vi "Dashboard Main.vi"() -> ()   [LabVIEW 2012]
uses:
  <vilib>/event_ctls.llb/eventvkey.ctl
  <vilib>/Utility/config.llb/Read Key (String).vi
  <vilib>/Utility/config.llb/Read Key (I32).vi
  <vilib>/Utility/config.llb/Write Key (String).vi
  <vilib>/Utility/config.llb/Write Key (I32).vi
  <vilib>/Utility/config.llb/NI_LVConfig.lvlib
panel:
  out "Mode":T1(ring)=enum."Auto Disabled"
  in  "Viewer":enum32{"Camera Image", "Variables"}(tab)
  out "Mbps":dbl format="%#.1g"
  in  "Enable":bool=TRUE
  in  "DB Camera Config":bool
  out "Mbps":bool
  out "fps":dbl format="%#.1g"
  out "Image Error Message":string="Timeout in Camera Communications"
  out "Camera Image":T2(plugin-control)
  out "Camera Image 2":T2(plugin-control)
  in  "Camera Settings":T3={"Frame Rate"=15, "Compression"=30, "Size"=1} {"Frame Rate" scale=1.0..30.0; "Size" items=["640x480", "320x240", "160x120"]}
  out "Camera IP 2":string
  out "Camera IP":string
  out "fps 2":dbl format="%#.1g"
  out "Mbps 2":dbl format="%#.1g"
  in  "Enable 2":bool=TRUE
  in  "FR":i32=15
  out "Tree":string(tree)
  in  "Dashboard Tab":enum32{"Operation", "Test", "Checklist"}(tab)
  in  "Slider":dbl(slide) scale=0.0..100.0 scale format="%#_3g"
  in  "On/Off":bool caption="Solenoid"
  in  "Test Name":u16(ring) items=["Select the test to run...", "Example Test", "-------------------------------", "List of tests is built in robot code.", "Replace with your own automated tests."]
  in  "Test Tree":string(tree)
  in  "Motor":cluster{"Value":dbl, "Enable":bool} {"Value" scale=-1.0..1.0 scale format="%#_3g"}
  out "Progress":T4 {"Test Progress" scale=0.0..100.0}
  in  "Rev/Fwd":cluster{"Forward":bool, "Reverse":bool}
  in  "Ring":u16(ring) items=["Auto", "Fixed indoor", "Fixed outdoor 1", "Fixed outdoor 2", "Fixed fluorescent 1", "Fixed fluorescent 2", "Hold current"]
  in  "Listbox":i32(listbox)
  out "Robot IP":string
  out "Battery Value":dbl(slide) scale=0.0..14.0 scale format="%#_2e"
  out "Battery":sgl(graph)
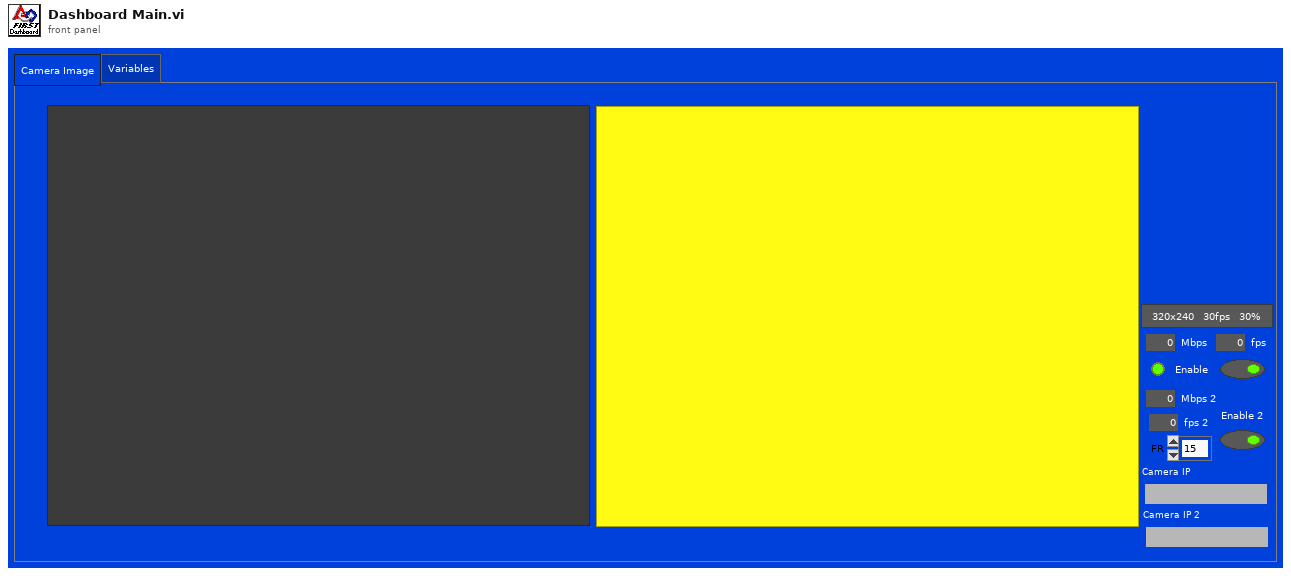
[diagram p1: front panel]
types:
  T1 = enum8{"Tele-Op Disabled", "Tele-Op Enabled", "Auto Disabled", "Auto Enabled", "Test Disabled", "Test Enabled", ""}
  T2 = typedef "IMAQ Image.ctl" = refnum<image>
  T3 = cluster{"Frame Rate":i32, "Compression":i32, "Size":u16}
  T4 = cluster{"Test Progress":u8, "Test Progress Text":string}
  T5 = typedef "Image Type" = u32
  T6 = cluster{"Competition mode":bool, "Robot Link":bool, "Autonomous":bool, "Enabled":bool, "E-Stop":bool, "Simulated":bool, "TestMode":bool, "Docked Window":bool}
  T7 = typedef "LVRectTypeDef.ctl" = cluster{"Left":i16, "Top":i16, "Right":i16, "Bottom":i16}
  T8 = typedef "NI_LVConfig.lvlib/Config Data RefNum.ctl" = refnum<k1>
  T9 = typedef "eventvkey.ctl" = enum16{"ASCII", "Enter", "Return", "Shift", "Ctrl", "Alt", "Cmd", "Opt", "Caps", "NumLock", "Clear", "Break", "Up", "Down", "Left", "Right", "Insert", "Delete", "Home", "End", "PageUp", "PageDown", "Escape", "Help", "Pause", "ScrollLock", "F1", "F2", "F3", "F4", "F5", "F6", "F7", "F8", "F9", "F10", "F11", "F12", "F13", "F14", "F15", "F16", "F17", "F18", "F19", "F20", "F21", "F22", "F23", "F24", "Play", "VolumeUp", "VolumeDown", "Mute", "Two Byte Char"}
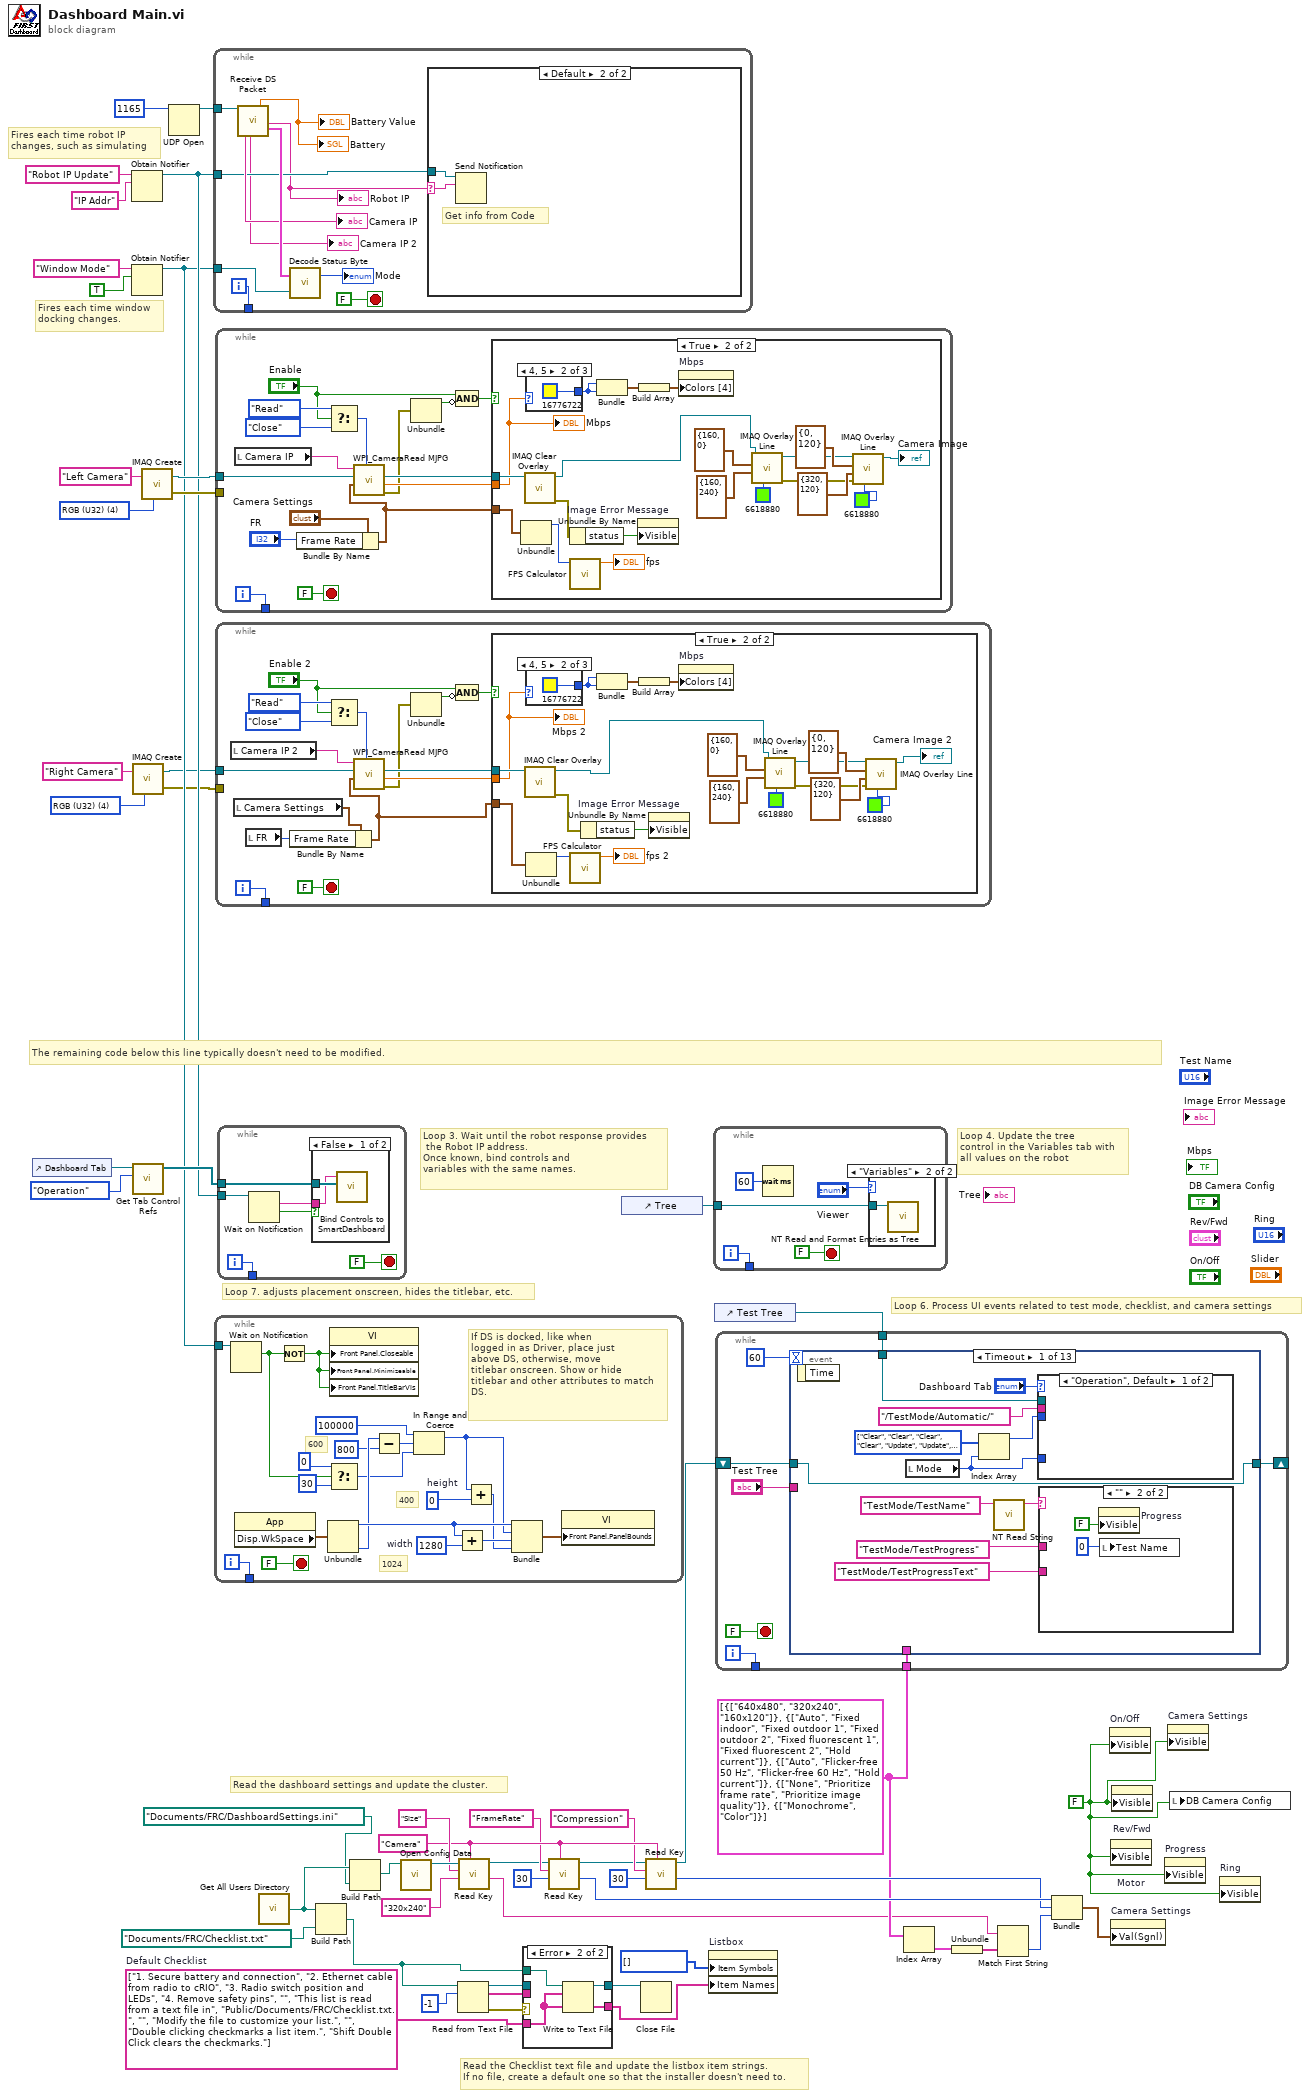
[diagram p0: block diagram]
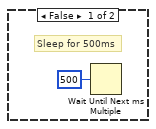
[diagram p2: hidden frame]
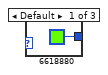
[diagram p3: hidden frame]
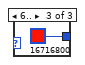
[diagram p4: hidden frame]
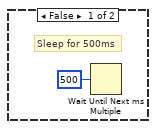
[diagram p6: hidden frame]
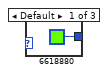
[diagram p7: hidden frame]
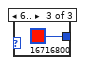
[diagram p8: hidden frame]
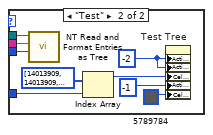
[diagram p10: hidden frame]
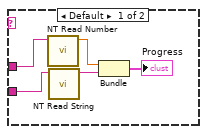
[diagram p11: hidden frame]
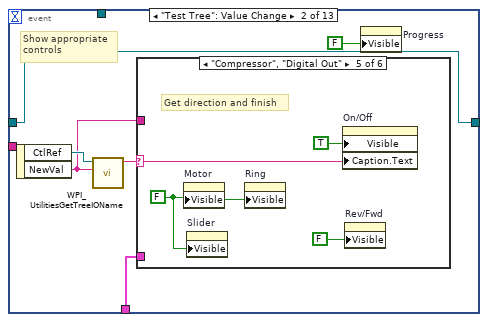
[diagram p12: hidden frame]
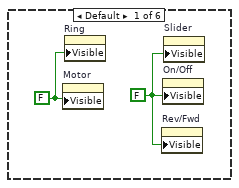
[diagram p13: hidden frame]
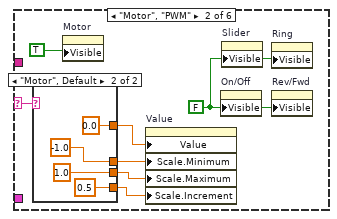
[diagram p14: hidden frame]
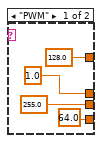
[diagram p15: hidden frame]
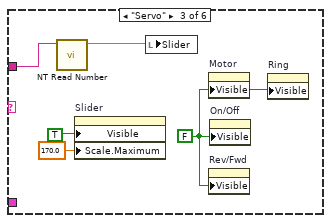
[diagram p16: hidden frame]
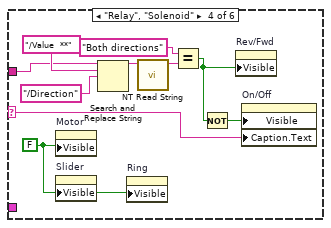
[diagram p17: hidden frame]
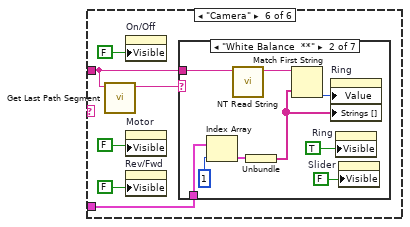
[diagram p18: hidden frame]
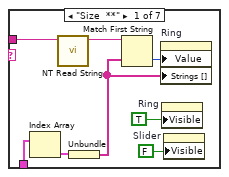
[diagram p19: hidden frame]
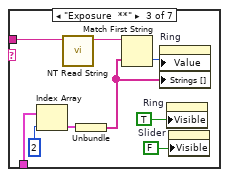
[diagram p20: hidden frame]
diagram:
  w3 = T5 4 items=["Grayscale (U8)", "Grayscale (I16)", "Grayscale (SGL)", "Complex (CSG)", "RGB (U32)", "HSL (U32)", "RGB (U64)"] ("Image Type")
  w25 = "Camera"
  w17 = cluster{string[]}[] [{["640x480", "320x240", "160x120"]}, {["Auto", "Fixed indoor", "Fixed outdoor 1", "Fixed outdoor 2", "Fixed fluorescent 1", "Fixed fluorescent 2", "Hold current"]}, {["Auto", "Flicker-free 50 Hz", "Flicker-free 60 Hz", "Hold current"]}, {["None", "Prioritize frame rate", "Prioritize image quality"]}, {["Monochrome", "Color"]}]
  w33 = string[] ["1. Secure battery and connection", "2. Ethernet cable from radio to cRIO", "3. Radio switch position and LEDs", "4. Remove safety pins", "", "This list is read from a text file in", "Public/Documents/FRC/Checklist.txt.", "", "Modify the file to customize your list.", "", "Double clicking checkmarks a list item.", "Shift Double Click clears the checkmarks."]  # Default Checklist
  w31 = FALSE ("Visible")
  w52 = T5 4 items=["Grayscale (U8)", "Grayscale (I16)", "Grayscale (SGL)", "Complex (CSG)", "RGB (U32)", "HSL (U32)", "RGB (U64)"] ("Image Type")
  # "Fires each time robot IP\nchanges, such as simulating"
  # "Fires each time window\ndocking changes."
  # "Read the Checklist text file and update the listbox item strings.\nIf no file, create a default one so that the installer doesn't need to."
  # "The remaining code below this line typically doesn't need to be modified."
  # "Loop 6. Process UI events related to test mode, checklist, and camera settings"
  # "Read the dashboard settings and update the cluster."
  # "Loop 4. Update the tree\ncontrol in the Variables tab with\nall values on the robot"
  # "Loop 3. Wait until the robot response provides\n the Robot IP address.\nOnce known, bind controls and\nvariables with the same names."
  # "Loop 7. adjusts placement onscreen, hides the titlebar, etc."
  n1 = control-ref of="Dashboard Tab"() -> (w47:refnum<vi>)
  n2 = Obtain Notifier(name (unnamed)="Robot IP Update", notification data type="IP Addr" ("name (unnamed)")) -> (notifier out=w44:refnum<notifier>)  [unwired: 2 in, 2 out]
  n3 = Obtain Notifier(name (unnamed)="Window Mode", notification data type=TRUE) -> (notifier out=w37:refnum<notifier>)  [unwired: 2 in, 2 out]
  n4 = call "IMAQ Create"("Image Name"="Right Camera", "Image Type"=w3) -> ("New Image"=w2:T2, "error out"=w1:errorcluster)  [unwired: 2 in, 1 out]
  n5 = call <vilib>:"Get Tab Control Refs.vi"("Page Index"=enum32{"Operation", "Test"}."Operation" ("Dashboard Tab"), "TabControl in"=w47) -> ("ControlsOnPage"=w48:refnum<vi>[])  [unwired: 9 in]
  n6 = call "IMAQ Create"("Image Name"="Left Camera", "Image Type"=w52) -> ("New Image"=w50:T2, "error out"=w49:errorcluster)  [unwired: 2 in, 1 out]
  n7 = UDP Open(11:u16 1165 ("port")) -> (port=w53:refnum<k16>)  [unwired: 2 in, 4 out]
  n8 = while {
    tunnel: w53 -> [w63]
    tunnel: w44 -> [w57]
    tunnel: w37 -> [w61]
    tunnel: [w58] -> _
    i -> [w58]
    stop <- FALSE stop-if-true
    n9 = call "Receive DS Packet.vi"("Recv Socket"=w63) -> ("Camera IP Address"=→"Camera IP":string, "Camera IP Address 2"=→"Camera IP 2":string, "Battery"=→"Battery" →"Battery Value":sgl, "Robot IP Address"=w56:string, "Status"=w64:T6)  [unwired: 8 in, 6 out]
    "Robot IP" <- w56
    n10 = call "Decode Status Byte.vi"("Window Mode Notifier"=w61, "Status"=w64) -> ("Mode"=→"Mode":T1)  [unwired: 1 out]
    n11 = case shown="Default" w56 {
      selector: w56 -> [_ w66]
      tunnel: w57 -> [_ w67]
      frame "0.0.0.0" {
        # "Robot not responding, don't poll the variables"
      }
      frame Default {
        # "Get info from Code"
        n12 = Send Notification(notification=w66, notifier=w67) -> ()  [unwired: 1 in, 2 out]
      }
    }
  }
  n13 = while {
    tunnel: w37 -> [w86]
    tunnel: [w84] -> _
    i -> [w84]
    stop <- FALSE stop-if-true
    w76 = 1280  # width
    w79 = 0  # height
    # "600"
    # "1024"
    # "400"
    # "If DS is docked, like when\nlogged in as Driver, place just\nabove DS, otherwise, move\ntitlebar onscreen. Show or hide\ntitlebar and other attributes to match\nDS."
    n14 = Wait on Notification(notifier=w86) -> (notification=w71:bool)  [unwired: 3 in, 3 out]
    n15 = property class="App"() -> ("Disp.WkSpace"=w82:T7)  [unwired: 2 in, 2 out]
    n16 = Not(x=w71) -> (.not. x?=w85:bool)
    n17 = Unbundle(w82) -> ("Left"=w80:i16, "Bottom"=w77:i16)  [unwired: 2 out]
    n18 = Select(t=0, s=w71, f=30) -> (s? t:f=w70:i32)
    n19 = property class="VI"("Front Panel.Closeable"=w85, "Front Panel.Minimizeable"=w85, "Front Panel.TitleBarVis"=w85) -> ()  [unwired: 2 in, 2 out]
    n20 = Subtract(x=w77, y=800) -> (x-y=w74:i32)
    n21 = In Range and Coerce(upper limit=100000, x=w74, lower limit=w70) -> (coerced(x)=w68:i32)  [unwired: 1 out]
    n22 = Add(x=w80, y=w76) -> (x+y=w81:i32)
    n23 = Add(x=w68, y=w79) -> (x+y=w78:i32)
    n24 = Bundle("Left"=w80, w68, w81, w78) -> (w83:cluster{"Left":i16, i32, i32, i32})  [unwired: 1 out]
    n25 = property class="VI"("Front Panel.PanelBounds"=w83) -> ()  [unwired: 2 in, 2 out]
  }
  n26 = while {
    tunnel: w50 -> [w100]
    tunnel: w49 -> [_]
    tunnel: [w102] -> _
    i -> [w102]
    stop <- FALSE stop-if-true
    n27 = local read "Camera IP"() -> (w101:string)
    n28 = Bundle By Name(cluster="Camera Settings", "Frame Rate"="FR") -> (w88:T3)
    n29 = Select(t=enum16{"Read", "Reopen", "Close"}."Read" ("Operation"), s="Enable", f=enum16{"Read", "Reopen", "Close"}."Close" ("Operation")) -> (s? t:f=w95:enum16{"Read", "Reopen", "Close"})
    n30 = call <vilib>:"WPI_CameraRead MJPG.vi"("Operation"=w95, "Camera Settings"=w88, "Image"=w100, "address"=w101) -> ("error out"=w94:errorcluster, "Bandwidth (kbps)"=w98:dbl, "Image Out"=w99:T2)  [unwired: 5 in]
    n31 = Unbundle(w94) -> ("status"=w92:bool)  [unwired: 2 out]
    n32 = Compound Arithmetic op=AND("Enable", invert w92) -> (w91:bool)
    n33 = case shown="True" w91 {
      tunnel: w88 -> [_ w116]
      tunnel: w99 -> [_ w119]
      tunnel: w98 -> [_ w118]
      frame False {
        # "Sleep for 500ms"
        n34 = Wait Until Next ms Multiple(millisecond multiple=u32 500) -> ()  [unwired: 1 out]
      }
      frame True {
        n35 = Unbundle(w116) -> ("Frame Rate"=w107:i32)  [unwired: 2 out]
        n36 = call "IMAQ Clear Overlay"("Image"=w119) -> ("error out"=w123:errorcluster, "Image Out"=w108:T2)  [unwired: 2 in, 7 out]
        n37 = case shown="4, 5" w118 {
          tunnel: [u32 6618880 ("Color Box") u32 16776722 ("Color Box") u32 16716800 ("Color Box")] -> w120
          frame Default {
          }
          frame 4, 5 {
          }
          frame 6.. {
          }
        }
        n38 = Unbundle By Name(w123) -> ("status"=w124:bool)
        n39 = call "FPS Calculator.vi"("Average Count"=w107) -> ("fps"=→"fps":dbl)  [unwired: 10 in]
        n40 = Bundle("Color Box"=w120, "Color Box"=w120) -> (w122:cluster{"Color Box":u32, "Color Box":u32})  [unwired: 1 out]
        n41 = property on="Image Error Message" class="Str"("Visible"=w124) -> ()  [unwired: 2 in, 2 out]
        n42 = Build Array(w122) -> (w121:cluster{"Color Box":u32, "Color Box":u32}[])
        n43 = property on="Mbps" class="Bool (strict)"("Colors [4]"=w121) -> ()  [unwired: 2 in, 2 out]
        n44 = call "IMAQ Overlay Line"("Color"=u32 6618880, "End Point"=cluster{"X":i32, "Y":i32} {"X"=160, "Y"=240}, "Start Point"=cluster{"X":i32, "Y":i32} {"X"=160, "Y"=0}, "Image"=w108) -> ("error out"=w113:errorcluster, "Image Out"=w112:T2)  [unwired: 6 in]
        n45 = call "IMAQ Overlay Line"("Color"=u32 6618880, "error in (no error)"=w113, "End Point"=cluster{"X":i32, "Y":i32} {"X"=320, "Y"=120}, "Start Point"=cluster{"X":i32, "Y":i32} {"X"=0, "Y"=120}, "Image"=w112) -> ("Image Out"=→"Camera Image":T2)  [unwired: 5 in, 1 out]
        "Mbps" <- w118
      }
    }
  }
  n46 = while {
    tunnel: w2 -> [w140]
    tunnel: [w142] -> _
    tunnel: w1 -> [_]
    i -> [w142]
    stop <- FALSE stop-if-true
    n47 = local read "Camera IP 2"() -> (w141:string)
    n48 = local read "Camera Settings"() -> (w129:T3)
    n49 = local read "FR"() -> (w130:i32)
    n50 = Bundle By Name(cluster=w129, "Frame Rate"=w130) -> (w128:T3)
    n51 = Select(t=enum16{"Read", "Reopen", "Close"}."Read" ("Operation"), s="Enable 2", f=enum16{"Read", "Reopen", "Close"}."Close" ("Operation")) -> (s? t:f=w135:enum16{"Read", "Reopen", "Close"})
    n52 = call <vilib>:"WPI_CameraRead MJPG.vi"("Operation"=w135, "Camera Settings"=w128, "Image"=w140, "address"=w141) -> ("error out"=w134:errorcluster, "Bandwidth (kbps)"=w138:dbl, "Image Out"=w139:T2)  [unwired: 5 in]
    n53 = Unbundle(w134) -> ("status"=w132:bool)  [unwired: 2 out]
    n54 = Compound Arithmetic op=AND("Enable 2", invert w132) -> (w131:bool)
    n55 = case shown="True" w131 {
      tunnel: w128 -> [_ w156]
      tunnel: w139 -> [_ w159]
      tunnel: w138 -> [_ w158]
      frame False {
        # "Sleep for 500ms"
        n56 = Wait Until Next ms Multiple(millisecond multiple=u32 500) -> ()  [unwired: 1 out]
      }
      frame True {
        n57 = call "IMAQ Clear Overlay"("Image"=w159) -> ("error out"=w163:errorcluster, "Image Out"=w146:T2)  [unwired: 2 in, 7 out]
        n58 = case shown="4, 5" w158 {
          tunnel: [u32 6618880 ("Color Box") u32 16776722 ("Color Box") u32 16716800 ("Color Box")] -> w160
          frame Default {
          }
          frame 4, 5 {
          }
          frame 6.. {
          }
        }
        n59 = Unbundle(w156) -> ("Frame Rate"=w155:i32)  [unwired: 2 out]
        n60 = call "FPS Calculator.vi"("Average Count"=w155) -> ("fps"=→"fps 2":dbl)  [unwired: 10 in]
        n61 = Unbundle By Name(w163) -> ("status"=w164:bool)
        n62 = Bundle("Color Box"=w160, "Color Box"=w160) -> (w162:cluster{"Color Box":u32, "Color Box":u32})  [unwired: 1 out]
        n63 = Build Array(w162) -> (w161:cluster{"Color Box":u32, "Color Box":u32}[])
        n64 = property on="Image Error Message" class="Str"("Visible"=w164) -> ()  [unwired: 2 in, 2 out]
        n65 = property on="Mbps" class="Bool (strict)"("Colors [4]"=w161) -> ()  [unwired: 2 in, 2 out]
        n66 = call "IMAQ Overlay Line"("Color"=u32 6618880, "End Point"=cluster{"X":i32, "Y":i32} {"X"=160, "Y"=240}, "Start Point"=cluster{"X":i32, "Y":i32} {"X"=160, "Y"=0}, "Image"=w146) -> ("error out"=w152:errorcluster, "Image Out"=w151:T2)  [unwired: 6 in]
        n67 = call "IMAQ Overlay Line"("Color"=u32 6618880, "error in (no error)"=w152, "End Point"=cluster{"X":i32, "Y":i32} {"X"=320, "Y"=120}, "Start Point"=cluster{"X":i32, "Y":i32} {"X"=0, "Y"=120}, "Image"=w151) -> ("Image Out"=→"Camera Image 2":T2)  [unwired: 5 in, 1 out]
        "Mbps 2" <- w158
      }
    }
  }
  n68 = while {
    tunnel: w48 -> [w173]
    tunnel: w44 -> [w170]
    tunnel: [w168] -> _
    i -> [w168]
    stop <- FALSE stop-if-true
    n69 = Wait on Notification(notifier=w170) -> (notification=w169:string, timed out?=w171:bool)  [unwired: 3 in, 2 out]
    n70 = case shown="False" w171 {
      tunnel: w173 -> [w175 _]
      tunnel: w169 -> [w174 _]
      frame False {
        n71 = call <vilib>:"Bind Controls to SmartDashboard.vi"("Bound Control Refs"=w175, "Server IP Address"=w174) -> ()  [unwired: 10 in]
      }
      frame True {
      }
    }
  }
  n72 = call "Get All Users Directory.vi"() -> ("All User Path"=w30:path)
  n73 = Build Path(base path=w30, name or relative path=path "Documents/FRC/Checklist.txt") -> (appended path=w34:path)
  n74 = Build Path(base path=w30, name or relative path=path "Documents/FRC/DashboardSettings.ini") -> (appended path=w29:path)
  n75 = call <vilib>:"Open Config Data.vi"("configuration file path"=w29) -> ("refnum"=w28:T8)  [unwired: 8 in, 2 out]
  n76 = Read from Text File(file (use dialog)=w34, count=-1 ("timeout ms (25000)")) -> (refnum out=w12:refnum<file>, text=w35:string[], error out=w36:errorcluster)  [unwired: 2 in, 1 out]
  n77 = call-poly <vilib>:"Read Key.vi"("section"=w25, "default value"="320x240", "key"="Size", "refnum"=w28) -> ("value"=w15:string, "refnum out"=w10:T8)  [unwired: 2 in, 4 out]
  n78 = case shown="Error" w36 {
    tunnel: w35 -> [w177 _]
    tunnel: [w177 w179] -> w32
    tunnel: w33 -> [_ w179]
    tunnel: w34 -> [_ w180]
    tunnel: [w176 w178] -> w11
    tunnel: w12 -> [w176 _]
    frame No Error {
    }
    frame Error {
      n79 = Write to Text File(file (use dialog)=w180, text=w179) -> (refnum out=w178:refnum<file>)  [unwired: 2 in, 2 out]
    }
  }
  n80 = call-poly <vilib>:"Read Key.vi"("section"=w25, "default value"=30, "key"="FrameRate", "refnum"=w10) -> ("value"=w20:i32, "refnum out"=w9:T8)  [unwired: 1 in, 5 out]
  n81 = control-ref of="Tree"() -> (w6:refnum<vi>)
  n82 = Close File(refnum=w11) -> ()  [unwired: 1 in, 2 out]
  n83 = call-poly <vilib>:"Read Key.vi"("section"=w25, "default value"=30, "key"="Compression", "refnum"=w9) -> ("value"=w19:i32, "refnum out"=w7:T8)  [unwired: 1 in, 5 out]
  n84 = property on="Listbox" class="LstBox (strict)"("Item Symbols"=i32[] [], "Item Names"=w32) -> ()  [unwired: 2 in, 2 out]
  n85 = while {
    tunnel: [w182] -> _
    tunnel: w6 -> [w181]
    i -> [w182]
    stop <- FALSE stop-if-true
    n86 = Wait (ms)(milliseconds to wait=u32 60) -> ()  [unwired: 1 out]
    n87 = case shown="\"Variables\"" "Viewer" {
      tunnel: w181 -> [_ w186]
      frame Default {
      }
      frame "Variables" {
        n88 = call <vilib>:"NT Read and Format Entries as Tree.vi"("Tree Refnum"=w186) -> ()  [unwired: 9 in, 2 out]
      }
    }
  }
  n89 = control-ref of="Test Tree"() -> (w5:refnum<vi>)
  n90 = while {
    tunnel: w17 -> [w191]
    shift-right: [w190] -> _
    shift-left: w7 -> [w189]
    tunnel: [w188] -> _
    tunnel: w5 -> [w187]
    i -> [w188]
    stop <- FALSE stop-if-true
    n91 = event shown="[0] Timeout" {
      selector: _ -> [_ _ _ _ _ _ _ _ _ _ _ _ _]
      dyn-events: _ -> [_ _ _ _ _ _ _ _ _ _ _ _ _]
      timeout: u32 60 ("milliseconds to wait") -> [_ _ _ _ _ _ _ _ _ _ _ _ _]
      tunnel: w187 -> [w201 _ _ _ _ _ _ _ _ _ _ _ _]
      tunnel: "Test Tree" -> [_ _ _ _ _ _ _ _ w395 w403 w405 w409 w417]
      tunnel: w191 -> [_ w223 _ _ _ _ w359 w389 _ _ _ _ _]
      tunnel: [w195 w222 _ w325 w333 w345 w358 w382 w394 w401 w404 w408 w416] -> w190
      tunnel: w189 -> [w195 w222 _ w325 w333 w345 w357 w382 w394 w401 w404 w408 w416]
      event Timeout {
        w200 = enum16{"Update", "Clear"}[] [enum."Clear", enum."Clear", enum."Clear", enum."Clear", enum."Update", enum."Update", enum."Clear"] items=["Update", "Clear"]
        n92 = event-data() -> ()  [unwired: 1 in, 1 out]
        n93 = local read "Mode"() -> (w198:T1)
        n94 = Index Array(array=w200, index=w198) -> (element=w199:enum16{"Update", "Clear"})
        n95 = call <vilib>:"NT Read String.vi"("Name"="TestMode/TestName") -> ("String"=w204:string)  [unwired: 9 in, 1 out]
        n96 = case shown="\"Operation\", Default" "Dashboard Tab" {
          tunnel: w201 -> [_ w214]
          tunnel: "/TestMode/Automatic/" ("Name Pattern") -> [_ w213]
          tunnel: w199 -> [_ w212]
          tunnel: w198 -> [_ w210]
          frame "Operation", Default {
          }
          frame "Test" {
            w209 = -2 ("Active Item:Row Number")
            n97 = call <vilib>:"NT Read and Format Entries as Tree.vi"("Operation"=w212, "Name Pattern"=w213, "Tree Refnum"=w214) -> ()  [unwired: 7 in, 2 out]
            n98 = Index Array(array=u32[] [14013909, 14013909, 14013909, 14013909, 14013909, 16777215, 14013909], index=w210) -> (element=w208:u32)
            n99 = property on="Test Tree" class="Tree (strict)"("Active Item Row Number"=w209, "ActiveColNum"=w209, "CellBG"=w208, "Active Item Row Number"=-1 ("Active Item:Row Number"), "CellBG"=u32 5789784 ("Color Box")) -> ()  [unwired: 2 in, 2 out]
          }
        }
        n100 = case shown="\"\"" w204 {
          tunnel: "TestMode/TestProgress" ("Name") -> [w216 _]
          tunnel: "TestMode/TestProgressText" ("Name") -> [w215 _]
          frame Default {
            n101 = call <vilib>:"NT Read Number.vi"("Name"=w216) -> ("Numeric"=w217:dbl)  [unwired: 9 in, 1 out]
            n102 = call <vilib>:"NT Read String.vi"("Name"=w215) -> ("String"=w218:string)  [unwired: 9 in, 1 out]
            n103 = Bundle("Numeric"=w217, "String"=w218) -> (→"Progress":cluster{"Numeric":dbl, "String":string})  [unwired: 1 in]
          }
          frame "" {
            n104 = property on="Progress" class="Clust (strict)"("Visible"=FALSE) -> ()  [unwired: 2 in, 2 out]
            n105 = local write "Test Name"(u16 0) -> ()
          }
        }
      }
      event "Test Tree": Value Change {
        # "Show appropriate\ncontrols"
        n106 = event-data() -> ("CtlRef"=w226:refnum<vi>, "NewVal"=w224:string)  [unwired: 1 in]
        n107 = call <vilib>:"WPI_UtilitiesGetTreeIOName.vi"("NewVal"=w224, "TreeControl in"=w226) -> ("I/O Name"=w227:string)  [unwired: 9 in]
        n108 = case shown="\"Compressor\", \"Digital Out\"" w227 {
          selector: w227 -> [_ w234 _ w252 w261 _]
          tunnel: w224 -> [_ _ w249 w251 _ w268]
          tunnel: w223 -> [_ _ _ _ _ w267]
          frame Default {
            w229 = FALSE ("Visible")
            w228 = FALSE ("Visible")
            n109 = property on="Motor" class="Clust (strict)"("Visible"=w228) -> ()  [unwired: 2 in, 2 out]
            n110 = property on="Ring" class="Ring (strict)"("Visible"=w228) -> ()  [unwired: 2 in, 2 out]
            n111 = property on="Rev/Fwd" class="Clust (strict)"("Visible"=w229) -> ()  [unwired: 2 in, 2 out]
            n112 = property on="On/Off" class="Bool (strict)"("Visible"=w229) -> ()  [unwired: 2 in, 2 out]
            n113 = property on="Slider" class="Slide (strict)"("Visible"=w229) -> ()  [unwired: 2 in, 2 out]
          }
          frame "Motor", "PWM" {
            w235 = FALSE ("Visible")
            n114 = case shown="\"Motor\", Default" w234 {
              tunnel: [1.0 ("Value") -1.0 ("Value")] -> w233
              tunnel: [255.0 ("Value") 1.0 ("Value")] -> w232
              tunnel: [128.0 ("Value") 0.0 ("Value")] -> w231
              tunnel: [64.0 ("Value") 0.5 ("Value")] -> w230
              frame "PWM" {
              }
              frame "Motor", Default {
              }
            }
            n115 = property on="Motor" class="Clust (strict)"("Visible"=TRUE) -> ()  [unwired: 2 in, 2 out]
            n116 = property on="Value" class="Slide (strict)"("Value"=w231, "Scale.Minimum"=w233, "Scale.Maximum"=w232, "Scale.Increment"=w230) -> ()  [unwired: 2 in, 2 out]
            n117 = property on="On/Off" class="Bool (strict)"("Visible"=w235) -> ()  [unwired: 2 in, 2 out]
            n118 = property on="Slider" class="Slide (strict)"("Visible"=w235) -> ()  [unwired: 2 in, 2 out]
            n119 = property on="Ring" class="Ring (strict)"("Visible"=w235) -> ()  [unwired: 2 in, 2 out]
            n120 = property on="Rev/Fwd" class="Clust (strict)"("Visible"=w235) -> ()  [unwired: 2 in, 2 out]
          }
          frame "Servo" {
            w247 = FALSE ("Visible")
            n121 = call <vilib>:"NT Read Number.vi"("Name"=w249) -> ("Numeric"=w248:dbl)  [unwired: 9 in, 1 out]
            n122 = property on="Slider" class="Slide (strict)"("Visible"=TRUE, "Scale.Maximum"=170.0 ("Scale.Range:Maximum")) -> ()  [unwired: 2 in, 2 out]
            n123 = local write "Slider"(w248) -> ()
            n124 = property on="Motor" class="Clust (strict)"("Visible"=w247) -> ()  [unwired: 2 in, 2 out]
            n125 = property on="Rev/Fwd" class="Clust (strict)"("Visible"=w247) -> ()  [unwired: 2 in, 2 out]
            n126 = property on="On/Off" class="Bool (strict)"("Visible"=w247) -> ()  [unwired: 2 in, 2 out]
            n127 = property on="Ring" class="Ring (strict)"("Visible"=w247) -> ()  [unwired: 2 in, 2 out]
          }
          frame "Relay", "Solenoid" {
            w250 = FALSE ("Visible")
            n128 = property on="Motor" class="Clust (strict)"("Visible"=w250) -> ()  [unwired: 2 in, 2 out]
            n129 = property on="Slider" class="Slide (strict)"("Visible"=w250) -> ()  [unwired: 2 in, 2 out]
            n130 = Search and Replace String(input string=w251, search string="/Value  **", replace string="/Direction") -> (result string=w257:string)  [unwired: 5 in, 3 out]
            n131 = property on="Ring" class="Ring (strict)"("Visible"=w250) -> ()  [unwired: 2 in, 2 out]
            n132 = call <vilib>:"NT Read String.vi"("Name"=w257) -> ("String"=w255:string)  [unwired: 9 in, 1 out]
            n133 = Equal?(x="Both directions", y=w255) -> (x = y?=w253:bool)
            n134 = Not(x=w253) -> (.not. x?=w254:bool)
            n135 = property on="Rev/Fwd" class="Clust (strict)"("Visible"=w253) -> ()  [unwired: 2 in, 2 out]
            n136 = property on="On/Off" class="Bool (strict)"("Visible"=w254, "Caption.Text"=w252) -> ()  [unwired: 2 in, 2 out]
          }
          frame "Compressor", "Digital Out" {
            w260 = FALSE ("Visible")
            # "Get direction and finish"
            n137 = property on="Motor" class="Clust (strict)"("Visible"=w260) -> ()  [unwired: 2 in, 2 out]
            n138 = property on="Slider" class="Slide (strict)"("Visible"=w260) -> ()  [unwired: 2 in, 2 out]
            n139 = property on="Ring" class="Ring (strict)"("Visible"=w260) -> ()  [unwired: 2 in, 2 out]
            n140 = property on="On/Off" class="Bool (strict)"("Visible"=TRUE, "Caption.Text"=w261) -> ()  [unwired: 2 in, 2 out]
            n141 = property on="Rev/Fwd" class="Clust (strict)"("Visible"=FALSE) -> ()  [unwired: 2 in, 2 out]
          }
          frame "Camera" {
            n142 = call <vilib>:"Get Last Path Segment.vi"("String in"=w268) -> ("String out"=w269:string)  [unwired: 10 in]
            n143 = property on="On/Off" class="Bool (strict)"("Visible"=FALSE) -> ()  [unwired: 2 in, 2 out]
            n144 = property on="Motor" class="Clust (strict)"("Visible"=FALSE) -> ()  [unwired: 2 in, 2 out]
            n145 = property on="Rev/Fwd" class="Clust (strict)"("Visible"=FALSE) -> ()  [unwired: 2 in, 2 out]
            n146 = case shown="\"White Balance  **\"" w269 {
              tunnel: w268 -> [w275 w284 w293 w302 w311 _ w317]
              tunnel: w267 -> [w273 w281 w290 w299 w308 _ _]
              frame "Size  **" {
                n147 = Index Array(array=w273) -> (element=w272:cluster{string[]})  [unwired: 1 in]
                n148 = call <vilib>:"NT Read String.vi"("Name"=w275) -> ("String"=w274:string)  [unwired: 9 in, 1 out]
                n149 = Unbundle(w272) -> (w270:string[])
                n150 = Match First String(2:w270, 3:w274) -> (0:w271:i32)  [unwired: 1 out]
                n151 = property on="Ring" class="Ring (strict)"("Value"=w271, "Strings []"=w270) -> ()  [unwired: 2 in, 2 out]
                n152 = property on="Ring" class="Ring (strict)"("Visible"=TRUE) -> ()  [unwired: 2 in, 2 out]
                n153 = property on="Slider" class="Slide (strict)"("Visible"=FALSE) -> ()  [unwired: 2 in, 2 out]
              }
              frame "White Balance  **" {
                n154 = Index Array(array=w281, index=1) -> (element=w282:cluster{string[]})
                n155 = call <vilib>:"NT Read String.vi"("Name"=w284) -> ("String"=w283:string)  [unwired: 9 in, 1 out]
                n156 = Unbundle(w282) -> (w279:string[])
                n157 = Match First String(2:w279, 3:w283) -> (0:w278:i32)  [unwired: 1 out]
                n158 = property on="Ring" class="Ring (strict)"("Value"=w278, "Strings []"=w279) -> ()  [unwired: 2 in, 2 out]
                n159 = property on="Ring" class="Ring (strict)"("Visible"=TRUE) -> ()  [unwired: 2 in, 2 out]
                n160 = property on="Slider" class="Slide (strict)"("Visible"=FALSE) -> ()  [unwired: 2 in, 2 out]
              }
              frame "Exposure  **" {
                n161 = Index Array(array=w290, index=2) -> (element=w291:cluster{string[]})
                n162 = call <vilib>:"NT Read String.vi"("Name"=w293) -> ("String"=w292:string)  [unwired: 9 in, 1 out]
                n163 = Unbundle(w291) -> (w287:string[])
                n164 = Match First String(2:w287, 3:w292) -> (0:w288:i32)  [unwired: 1 out]
                n165 = property on="Ring" class="Ring (strict)"("Value"=w288, "Strings []"=w287) -> ()  [unwired: 2 in, 2 out]
                n166 = property on="Ring" class="Ring (strict)"("Visible"=TRUE) -> ()  [unwired: 2 in, 2 out]
                n167 = property on="Slider" class="Slide (strict)"("Visible"=FALSE) -> ()  [unwired: 2 in, 2 out]
              }
              frame "Exposure Priority  **" {
                n168 = Index Array(array=w299, index=3) -> (element=w300:cluster{string[]})
                n169 = call <vilib>:"NT Read String.vi"("Name"=w302) -> ("String"=w301:string)  [unwired: 9 in, 1 out]
                n170 = Unbundle(w300) -> (w296:string[])
                n171 = Match First String(2:w296, 3:w301) -> (0:w297:i32)  [unwired: 1 out]
                n172 = property on="Ring" class="Ring (strict)"("Value"=w297, "Strings []"=w296) -> ()  [unwired: 2 in, 2 out]
                n173 = property on="Ring" class="Ring (strict)"("Visible"=TRUE) -> ()  [unwired: 2 in, 2 out]
                n174 = property on="Slider" class="Slide (strict)"("Visible"=FALSE) -> ()  [unwired: 2 in, 2 out]
              }
              frame "Color Enable  **" {
                n175 = Index Array(array=w308, index=4) -> (element=w309:cluster{string[]})
                n176 = call <vilib>:"NT Read String.vi"("Name"=w311) -> ("String"=w310:string)  [unwired: 9 in, 1 out]
                n177 = Unbundle(w309) -> (w305:string[])
                n178 = Match First String(2:w305, 3:w310) -> (0:w306:i32)  [unwired: 1 out]
                n179 = property on="Ring" class="Ring (strict)"("Value"=w306, "Strings []"=w305) -> ()  [unwired: 2 in, 2 out]
                n180 = property on="Ring" class="Ring (strict)"("Visible"=TRUE) -> ()  [unwired: 2 in, 2 out]
                n181 = property on="Slider" class="Slide (strict)"("Visible"=FALSE) -> ()  [unwired: 2 in, 2 out]
              }
              frame Default {
                n182 = property on="Ring" class="Ring (strict)"("Visible"=FALSE) -> ()  [unwired: 2 in, 2 out]
                n183 = property on="Slider" class="Slide (strict)"("Visible"=FALSE) -> ()  [unwired: 2 in, 2 out]
              }
              frame "Brightness  **", "Color Level  **", "Compression  **", "FPS  **", "Sharpness  **" {
                n184 = call <vilib>:"NT Read Number.vi"("Name"=w317) -> ("Numeric"=w316:dbl)  [unwired: 9 in, 1 out]
                n185 = local write "Slider"(w316) -> ()
                n186 = property on="Slider" class="Slide (strict)"("Visible"=TRUE, "Scale.Maximum"=100.0 ("Scale.Range:Maximum")) -> ()  [unwired: 2 in, 2 out]
                n187 = property on="Ring" class="Ring (strict)"("Visible"=FALSE) -> ()  [unwired: 2 in, 2 out]
              }
            }
          }
        }
        n188 = property on="Progress" class="Clust (strict)"("Visible"=FALSE) -> ()  [unwired: 2 in, 2 out]
      }
      event "Test Name": Mouse Enter {
        # "Populate the ring with the list of tests"
        n189 = event-data() -> ()  [unwired: 1 in, 1 out]
        n190 = call <vilib>:"NT Read String Array.vi"("Name"="TestMode/TestList") -> ("String Array"=w324:string[])  [unwired: 9 in, 1 out]
        n191 = Build Array (concatenate)("Select the test to run...", w324) -> (w323:string[])
        n192 = property on="Test Name" class="Ring (strict)"("Strings []"=w323) -> ()  [unwired: 2 in, 2 out]
      }
      event "Test Name": Value Change {
        w326 = FALSE ("Visible")
        # "Tell the robot the test name to run"
        n193 = event-data() -> ("NewVal"=w330:u16)  [unwired: 1 in]
        n194 = property on="Test Name" class="Ring (strict)"() -> ("Strings []"=w331:string[])  [unwired: 2 in, 2 out]
        n195 = local write "Progress"(T4 {"Test Progress"=0, "Test Progress Text"=""} ("Progress")) -> ()
        n196 = Index Array(array=w331, index=w330) -> (element=w329:string)
        n197 = call <vilib>:"NT Write String.vi"("String"=w329, "Name"="TestMode/TestName") -> ()  [unwired: 9 in, 1 out]
        n198 = property on="Progress" class="Clust (strict)"("Visible"=TRUE) -> ()  [unwired: 2 in, 2 out]
        n199 = property on="Motor" class="Clust (strict)"("Visible"=w326) -> ()  [unwired: 2 in, 2 out]
        n200 = property on="Slider" class="Slide (strict)"("Visible"=w326) -> ()  [unwired: 2 in, 2 out]
        n201 = property on="On/Off" class="Bool (strict)"("Visible"=w326) -> ()  [unwired: 2 in, 2 out]
        n202 = property on="Rev/Fwd" class="Clust (strict)"("Visible"=w326) -> ()  [unwired: 2 in, 2 out]
        n203 = property on="Ring" class="Ring (strict)"("Visible"=w326) -> ()  [unwired: 2 in, 2 out]
      }
      event "Listbox": Double Click {
        n204 = event-data() -> ("PlatMods.Shift"=w334:bool, "Row"=w336:i32)  [unwired: 1 in]
        n205 = case shown="False" w334 {
          tunnel: w336 -> [w340 _]
          tunnel: 1 -> [w339 _]
          frame False {
            n206 = property on="Listbox" class="LstBox (strict)"() -> ("Item Symbols"=w338:i32[])  [unwired: 2 in, 2 out]
            n207 = Replace Array Subset(array=w338, new element=w339, index=w340) -> (w337:i32[])
            n208 = property on="Listbox" class="LstBox (strict)"("Item Symbols"=w337) -> ()  [unwired: 2 in, 2 out]
          }
          frame True {
            w341 = 0 ("Top Row")
            n209 = property on="Listbox" class="LstBox (strict)"() -> ("Number of Rows"=w343:u32)  [unwired: 2 in, 2 out]
            n210 = Initialize Array(0, w343) -> (w342:i32[])
            n211 = property on="Listbox" class="LstBox (strict)"("Top Row"=w341, "Value"=w341, "Item Symbols"=w342) -> ()  [unwired: 2 in, 2 out]
          }
        }
      }
      event "Listbox": Key Down {
        n212 = event-data() -> ("VKey"=w347:T9)  [unwired: 1 in]
        n213 = case shown="\"Left\", \"Right\"" w347 {
          selector: w347 -> [w352 _]
          tunnel: eventvkey."Left" ("VKey") -> [w350 _]
          frame "Left", "Right" {
            n214 = Equal?(x=w350, y=w352) -> (x = y?=w351:bool)
            n215 = Select(t=0, s=w351, f=1) -> (s? t:f=w353:i32)
            n216 = property on="Listbox" class="LstBox (strict)"() -> ("Item Symbols"=w356:i32[])  [unwired: 2 in, 2 out]
            n217 = Replace Array Subset(array=w356, new element=w353, index="Listbox") -> (w355:i32[])
            n218 = property on="Listbox" class="LstBox (strict)"("Item Symbols"=w355) -> ()  [unwired: 2 in, 2 out]
          }
          frame Default {
          }
        }
      }
      event "DB Camera Config": Value Change {
        n219 = event-data() -> ("NewVal"=w360:bool)  [unwired: 1 in]
        n220 = case shown="False" w360 {
          tunnel: w359 -> [w369 _]
          tunnel: [w362 w380] -> w358
          tunnel: w357 -> [w361 w380]
          frame False {
            w376 = "Camera"
            w379 = FALSE ("Visible")
            n221 = local read "Camera Settings"() -> (w368:T3)
            n222 = Index Array(array=w369) -> (element=w372:cluster{string[]})  [unwired: 1 in]
            n223 = Unbundle(w368) -> ("Frame Rate"=w367:i32, "Compression"=w366:i32, "Size"=w370:u16)
            n224 = Unbundle(w372) -> (w371:string[])
            n225 = Index Array(array=w371, index=w370) -> (element=w365:string)
            n226 = call-poly <vilib>:"Write Key.vi"("section"=w376, "value"=w365, "key"="Size", "refnum"=w361) -> ("refnum out"=w378:T8)  [unwired: 2 in, 5 out]
            n227 = call-poly <vilib>:"Write Key.vi"("section"=w376, "value"=w367, "key"="FrameRate", "refnum"=w378) -> ("refnum out"=w377:T8)  [unwired: 1 in, 6 out]
            n228 = property on="Camera Settings" class="Clust (strict)"("Visible"=w379) -> ()  [unwired: 2 in, 2 out]
            n229 = local write "DB Camera Config"(w379) -> ()
            n230 = call-poly <vilib>:"Write Key.vi"("section"=w376, "value"=w366, "key"="Compression", "refnum"=w377) -> ("refnum out"=w363:T8)  [unwired: 1 in, 6 out]
            n231 = call <vilib>:"Close Config Data.vi"("refnum"=w363) -> ("file path"=w364:path)  [unwired: 2 in, 8 out]
            n232 = call <vilib>:"Open Config Data.vi"("configuration file path"=w364) -> ("refnum"=w362:T8)  [unwired: 8 in, 2 out]
          }
          frame True {
            n233 = property on="Camera Settings" class="Clust (strict)"("Visible"=TRUE) -> ()  [unwired: 2 in, 2 out]
          }
        }
      }
      event "Camera Settings": Value Change {
        n234 = event-data() -> ("NewVal"=w393:T3)  [unwired: 1 in]
        n235 = Index Array(array=w389) -> (element=w388:cluster{string[]})  [unwired: 1 in]
        n236 = Unbundle(w393) -> ("Frame Rate"=w384:i32, "Compression"=w383:i32, "Size"=w386:u16)
        n237 = Unbundle(w388) -> (w387:string[])
        n238 = Index Array(array=w387, index=w386) -> (element=w385:string)
        n239 = Format Into String(format string="%s   %dfps   %d%%", w385, w384, w383) -> (resulting string=w390:string)  [unwired: 2 in, 1 out]
        n240 = Build Array(w390) -> (w391:string[])
        n241 = property on="DB Camera Config" class="Bool (strict)"("Strings [4]"=w391) -> ()  [unwired: 2 in, 2 out]
      }
      event "Motor.Enable": Value Change {
        n242 = event-data() -> ("NewVal"=w399:bool)  [unwired: 1 in]
        n243 = Unbundle("Motor") -> ("Value"=w398:dbl)  [unwired: 1 out]
        n244 = Select(t=w398, s=w399, f=0.0) -> (s? t:f=w396:dbl)
        n245 = call <vilib>:"NT Write Number.vi"("Numeric"=w396, "Name"=w395) -> ()  [unwired: 9 in, 1 out]
      }
      event "Slider": Value Change {
        n246 = event-data() -> ("NewVal"=w402:dbl)  [unwired: 1 in]
        n247 = call <vilib>:"NT Write Number.vi"("Numeric"=w402, "Name"=w403) -> ()  [unwired: 9 in, 1 out]
      }
      event "On/Off": Value Change {
        n248 = event-data() -> ("NewVal"=w407:bool)  [unwired: 1 in]
        n249 = Boolean To (0,1)(Boolean=w407) -> (0, 1=w406:i16)
        n250 = call <vilib>:"NT Write Number.vi"("Numeric"=w406, "Name"=w405) -> ()  [unwired: 9 in, 1 out]
      }
      event "Rev/Fwd": Value Change {
        n251 = event-data() -> ("NewVal.Forward"=w415:bool, "NewVal.Reverse"=w414:bool)  [unwired: 1 in]
        n252 = Boolean To (0,1)(Boolean=w415) -> (0, 1=w411:i16)
        n253 = Boolean To (0,1)(Boolean=w414) -> (0, 1=w413:i16)
        n254 = Negate(x=w413) -> (-x=w412:i16)
        n255 = Add(x=w411, y=w412) -> (x+y=w410:i16)
        n256 = call <vilib>:"NT Write Number.vi"("Numeric"=w410, "Name"=w409) -> ()  [unwired: 9 in, 1 out]
      }
      event "Ring": Value Change {
        n257 = event-data() -> ("NewVal"=w419:u16)  [unwired: 1 in]
        n258 = property on="Ring" class="Ring (strict)"() -> ("Strings []"=w420:string[])  [unwired: 2 in, 2 out]
        n259 = Index Array(array=w420, index=w419) -> (element=w418:string)
        n260 = call <vilib>:"NT Write String.vi"("String"=w418, "Name"=w417) -> ()  [unwired: 9 in, 1 out]
      }
    }
  }
  n261 = Index Array(array=w17) -> (element=w18:cluster{string[]})  [unwired: 1 in]
  n262 = Unbundle(w18) -> (w16:string[])
  n263 = Match First String(2:w16, 3:w15) -> (0:w14:i32)  [unwired: 1 out]
  n264 = Bundle("value"=w20, "value"=w19, "index"=w14) -> (w8:cluster{"value":i32, "value":i32, "index":i32})  [unwired: 1 out]
  n265 = property on="On/Off" class="Bool (strict)"("Visible"=w31) -> ()  [unwired: 2 in, 2 out]
  n266 = property on="Motor" class="Clust (strict)"("Visible"=w31) -> ()  [unwired: 2 in, 2 out]
  n267 = property on="Camera Settings" class="Clust (strict)"("Val(Sgnl)"=w8) -> ()  [unwired: 2 in, 2 out]
  n268 = property on="Rev/Fwd" class="Clust (strict)"("Visible"=w31) -> ()  [unwired: 2 in, 2 out]
  n269 = property on="Progress" class="Clust (strict)"("Visible"=w31) -> ()  [unwired: 2 in, 2 out]
  n270 = property on="Camera Settings" class="Clust (strict)"("Visible"=w31) -> ()  [unwired: 2 in, 2 out]
  n271 = local write "DB Camera Config"(w31) -> ()
  n272 = property on="Ring" class="Ring (strict)"("Visible"=w31) -> ()  [unwired: 2 in, 2 out]
